vi "PKG_IMC_WaitParamBit.vi"(4 "fifo":i32, 5 "axis":i32, 6 "timeout":i32, 7 "val":i16, 9 "bit":i16, 10 "paramloc":i16, 11 "Handle":u32) -> (2 "function return":i32, 3 "Handle out":u32)   [LabVIEW 2011, in "IMC_Pkg4xxx.lvlib"]
doc: "PKG_IMC_WaitParamBit(IMC_HANDLE Handle, short paramloc, short bit, short val, int timeout, int axis, int fifo);"
uses:
  IMC_Pkg4xxx.lvlib
  IMC_Pkg4xxx.dll
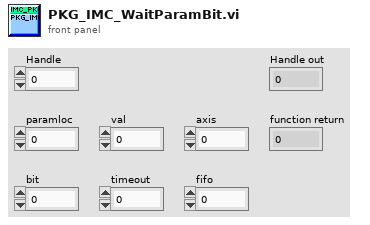
[diagram p1: front panel]
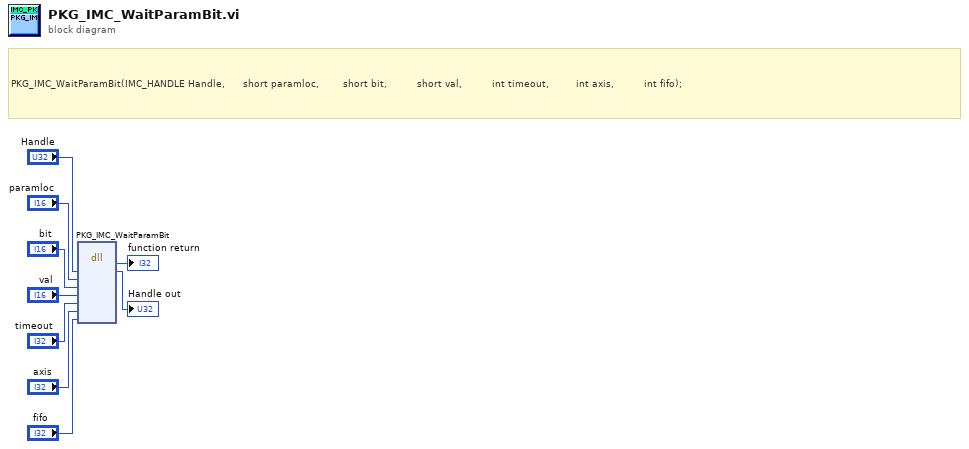
[diagram p0: block diagram]
diagram:
  # "PKG_IMC_WaitParamBit(IMC_HANDLE Handle,\t\t\t\t\t\tshort paramloc, \t\t\t\t\t\t\tshort bit, \t\t\t\t\t\t\t\t\tshort val, \t\t\t\t\t\t\t\t\tint timeout, \t\t\t\t\t\t\t\tint axis, \t\t\t\t\t\t\t\t\tint fifo);"
  n1 = dll-call lib="PTH1mabs F光盘刻录\niMC MotionIMCNet_V4.0IMCAppincLabviewIMC_PKG4xxxIMC_PKG4xxx\nIMC_Pkg4xxx.*" fn="PKG_IMC_WaitParamBit"("Handle"="Handle", "paramloc"="paramloc", "bit"="bit", "val"="val", "timeout"="timeout", "axis"="axis", "fifo"="fifo") -> (→"function return":i32, "Handle"=→"Handle out":u32)  [unwired: 9 in, 2 out]
